vi "Mean Time to Resolution.vi"(8 "error in (no error)":errorcluster, 11 "alarms in":refnum<class "NI SystemLink Alarm.lvclass">[](array[class])) -> (0 "error out":errorcluster, 1 "MTTR of inactive alarms (days)":dbl format="%#.2g", 2 "MTTR of inactive alarms (HH:MM:SS)":dbl format="%<%H:%M:%S>t", 3 "alarms out":refnum<class "NI SystemLink Alarm.lvclass">[](array[class]), 4 "MTTR Array":dbl[](array[numeric]) format="%<%H:%M:%S>t", 5 "# of resolved (inactive) alarms":i32)   [LabVIEW 2019, in "SystemLink Alarm KPIs.lvlib"]
uses:
  SystemLink Alarm KPIs.lvlib
  <vilib>/Skyline/Alarm/Class/NI SystemLink Alarm.lvclass
  <vilib>/Skyline/Alarm/Class/NI SystemLink Alarm.lvclass/NI SystemLink Alarm.ctl
  <vilib>/Skyline/Alarm/Class/Accessors/Read Acknowledged At.vi
  <vilib>/Skyline/Alarm/Class/Accessors/Read Active.vi
  <vilib>/Analysis/baseanly.llb/Mean (DBL).vi
  <vilib>/Skyline/Alarm/Class/Private/Ensure Alarm Information.vi
  <vilib>/Skyline/Alarm/Class/Accessors/Read Transitions.vi
  <vilib>/Skyline/Alarm/Library/Get Alarm Information.vi
  <vilib>/Analysis/NI_AALBase.lvlib
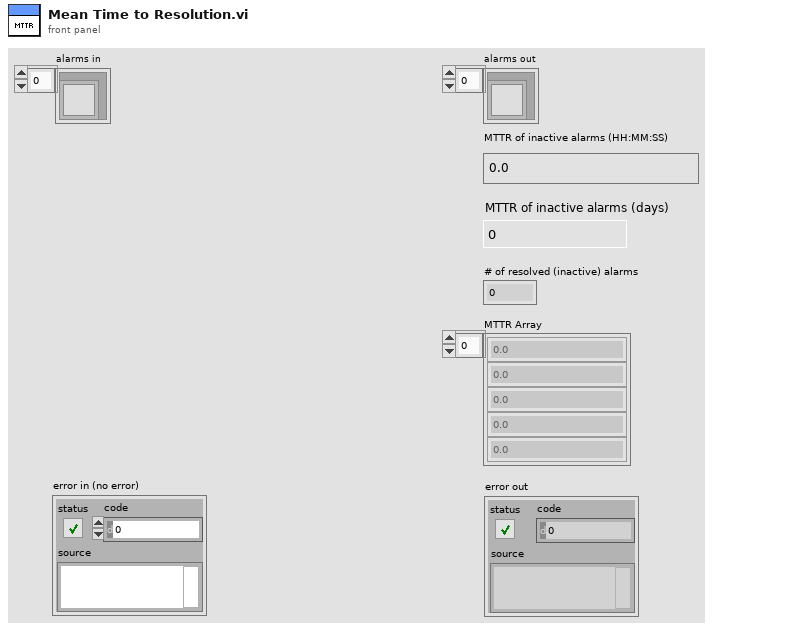
[diagram p1: front panel]
types:
  T1 = typedef "NI SystemLink Alarm Library.lvlib/Transition.ctl" = cluster{"type":T2, "severity level":T3, "condition":string, "occurred at":timestamp, "keywords":string[], "properties":T4[]}
  T2 = typedef "NI SystemLink Alarm Library.lvlib/Transition Type.ctl" = enum16{"Set", "Clear"}
  T3 = typedef "NI SystemLink Alarm Library.lvlib/Severity Level.ctl" = i32
  T4 = typedef "NI Skyline Utilities.lvlib/Property.ctl" = cluster{"key":string, "value":string}
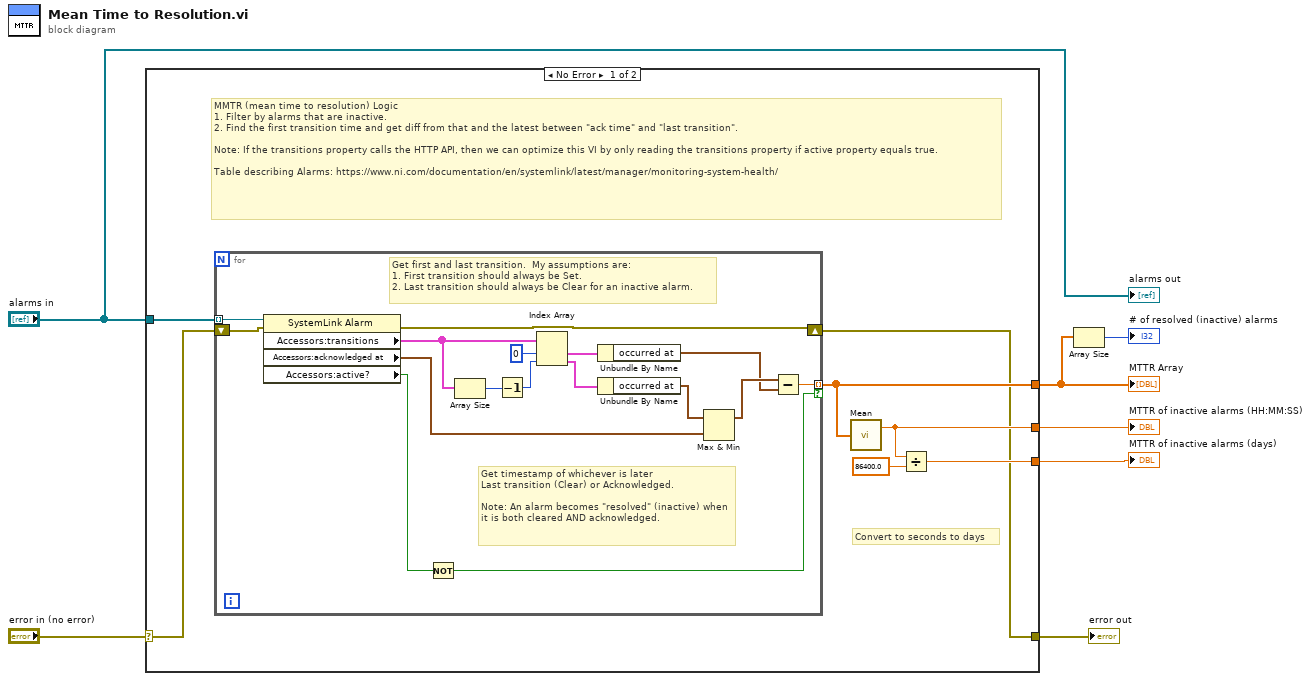
[diagram p0: block diagram]
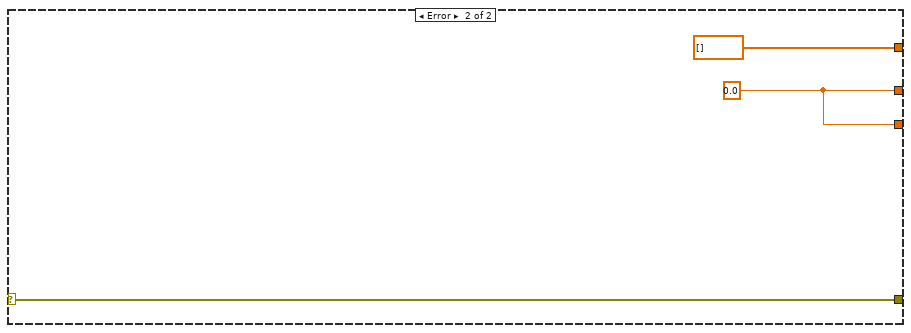
[diagram p2: hidden frame]
diagram:
  n1 = case shown="No Error" "error in (no error)" {
    selector: "error in (no error)" -> [w9 w31]
    tunnel: [w14 dbl[] []] -> w1
    tunnel: [w12 w32] -> w7
    tunnel: "alarms in" -> [w11 _]
    tunnel: [w10 w32] -> w5
    tunnel: [w8 w31] -> w3
    frame No Error {
      # "Convert to seconds to days"
      # "MMTR (mean time to resolution) Logic\n1. Filter by alarms that are inactive.\n2. Find the first transition time and get diff from that and the latest between \"ack time\" and \"last transition\".\n\nNote: If the transitions property calls the HTTP API, then we can optimize this VI by only reading the transitions property if active property equals true.\n\nTable describing Alarms: https://www.ni.com/documentation/en/systemlink/latest/manager/monitoring-system-health/"
      n2 = for {
        tunnel: w11 -> [w30] mode=indexing
        tunnel: [w19] -> w14 mode=indexing if=w15
        shift-right: [w17] -> w8
        shift-left: w9 -> [w18]
        # "Get timestamp of whichever is later\nLast transition (Clear) or Acknowledged.\n\nNote: An alarm becomes \"resolved\" (inactive) when it is both cleared AND acknowledged."
        # "Get first and last transition.  My assumptions are:\n1. First transition should always be Set.\n2. Last transition should always be Clear for an inactive alarm."
        n3 = property class="SystemLink Alarm"(reference=w30, error in=w18) -> (error out=w17:errorcluster, "Accessors:transitions"=w28:T1[], "Accessors:acknowledged at"=w22:timestamp, "Accessors:active?"=w16:bool)  [unwired: 1 out]
        n4 = Not(x=w16) -> (.not. x?=w15:bool)
        n5 = Array Size(array=w28) -> (size(s)=w27:i32)
        n6 = Decrement(x=w27) -> (x-1=w26:i32)
        n7 = Index Array(array=w28, index #1=0 ("index"), index #2=w26) -> (element #1=w25:T1, element #2=w24:T1)
        n8 = Unbundle By Name(w25) -> ("occurred at"=w20:timestamp)
        n9 = Unbundle By Name(w24) -> ("occurred at"=w23:timestamp)
        n10 = Max & Min(x=w23, y=w22) -> (max(x,y)=w21:timestamp)  [unwired: 1 out]
        n11 = Subtract(x=w21, y=w20) -> (x-y=w19:dbl)
      }
      n12 = call-poly <vilib>:"Mean.vi"("X"=w14) -> ("mean"=w10:dbl)  [unwired: 1 out]
      n13 = Divide(x=w10, y=86400.0) -> (x/y=w12:dbl)
    }
    frame Error {
      w32 = 0.0 ("mean")
    }
  }
  "MTTR Array" <- w1
  "MTTR of inactive alarms (HH:MM:SS)" <- w5
  "MTTR of inactive alarms (days)" <- w7
  "error out" <- w3
  n14 = Array Size(array=w1) -> (size(s)=→"# of resolved (inactive) alarms":i32)
  "alarms out" <- "alarms in"
